vi "fgt get power.vi"(8 "error in (no error)":errorcluster, 11 "controllerIndex":u16) -> (0 "error out":errorcluster, 3 "powerState":T1)   [LabVIEW 2020, in "fgt_SDK.lvlib"]
doc: "Get power information about a controller (such as Link, MFCS, Flowboard).\nNot all controllers support this functionality."
uses:
  fgt_SDK.lvlib
  TypeDefs/fgt_POWER.ctl
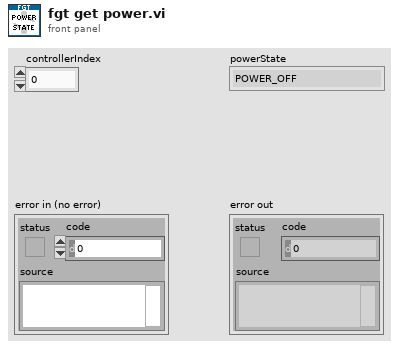
[diagram p1: front panel]
types:
  T1 = typedef "fgt_SDK.lvlib/fgt_POWER.ctl" = enum8{"POWER_OFF", "POWER_ON", "SLEEP"}
  T2 = typedef "fgt_SDK.lvlib/fgt_STATUS_INFO.ctl" = cluster{"InstrType":T3, "instrSN":u16, "errorCode":u8, "infoCode":u8, "detail":string}
  T3 = typedef "fgt_SDK.lvlib/fgt_INSTRUMENT_TYPE.ctl" = enum32{"None", "MFCS", "MFCS_EZ", "FRP", "LineUP", "IPS"}
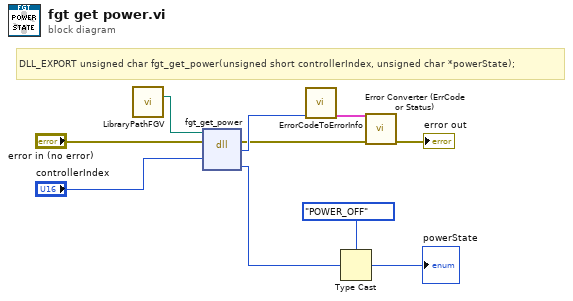
[diagram p0: block diagram]
diagram:
  # "DLL_EXPORT unsigned char fgt_get_power(unsigned short controllerIndex, unsigned char *powerState);"
  n1 = call "LibraryPathFGV.vi"() -> ("Path Out"=w1:path)  [unwired: 14 in, 1 out]
  n2 = dll-call lib="C:/Workspace/fgt-SDK/LabVIEW/dlls/fgt_SDK_*.*" fn="fgt_get_power"(path in=w1, error in="error in (no error)", "controllerIndex"="controllerIndex") -> (error out=w5:errorcluster, "return type"=w7:u8, "powerState"=w2:u8)  [unwired: 3 in, 1 out]
  n3 = call "ErrorCodeToErrorInfo.vi"("return type"=w7) -> ("StatusInfo"=w6:T2)  [unwired: 10 in]
  n4 = Type Cast(type=fgt_POWER."POWER_OFF" ("powerState"), x=w2) -> (*(type *) &x=→"powerState":T1)
  n5 = call "Error Converter (ErrCode or Status).vi"("error in (no error)"=w5, "StatusInfo"=w6) -> ("error out"=→"error out":errorcluster)  [unwired: 9 in]
